vi "WW_Spin_Analysis_V2.vi"(11 "路径":path) -> (3 "strArrayError":string[](array[string]))   [LabVIEW 2011]
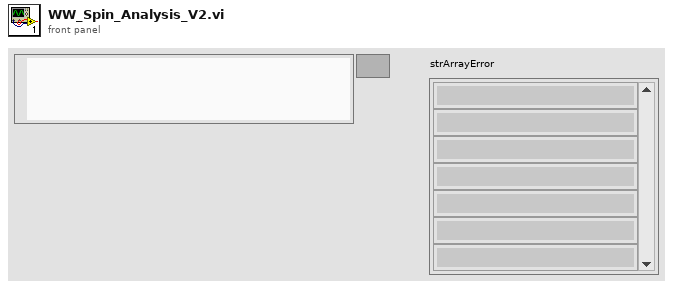
[diagram p1: front panel]
types:
  T1 = enum16{"RealTime", "WaterLevel", "WaterTemp", "AirTemp", "IPMTemp", "MotorActualRPM", "MotorTargetRPM", "FanActualRPM", "MemsSensorA", "MemsSensorB", "MemsSensorC", "WaterThermistorADC", "TouchSensor", "LeakageSensor", "DCLink", "IsDoorOpen", "IsTimeShort", "Progress", "Step", "TotalRemainTime", "StepRemainTime", "WeightSensingLowData", "WeightSensingResult", "ColdValve", "HotValve", "PreValve", "WaterShotValve", "BleachValve", "DryValve", "SteamValve", "SoftenerValve", "FilterValve", "IsDoorLocked", "SSRCommon", "MainRelay", "ACTUATOR2", "WaterDrainer", "CirculationPump", "WaterHeater", "DryHeater", "SteamHeater", "MotorDriveDirection", "IsDoubleDoorOpen", "IsDoubleDoorLock", "RunStateID", "PowerStateID", "SoundID", "ErrorCode", "OptionData", "MainVersion", "SUBVersion", "InverterVersion"}
  T2 = cluster{"mu32DrainIndex":u32, "mu32SpinIndex":u32, "mu32LooseInex":u32}
  T3 = cluster{"DrainTime":u32, "FinalSpinTime":u32, "LooseTime":u32, "SubTotalTime":u32}
  T4 = cluster{"Step1":cluster{"Speed":u32, "Time":u32}, "Step2":cluster{"Speed":u32, "Time":u32}, "Step3":cluster{"Speed":u32, "Time":u32}, "Untangle":cluster{"Speed":u32, "On":u32, "Off":u32}}
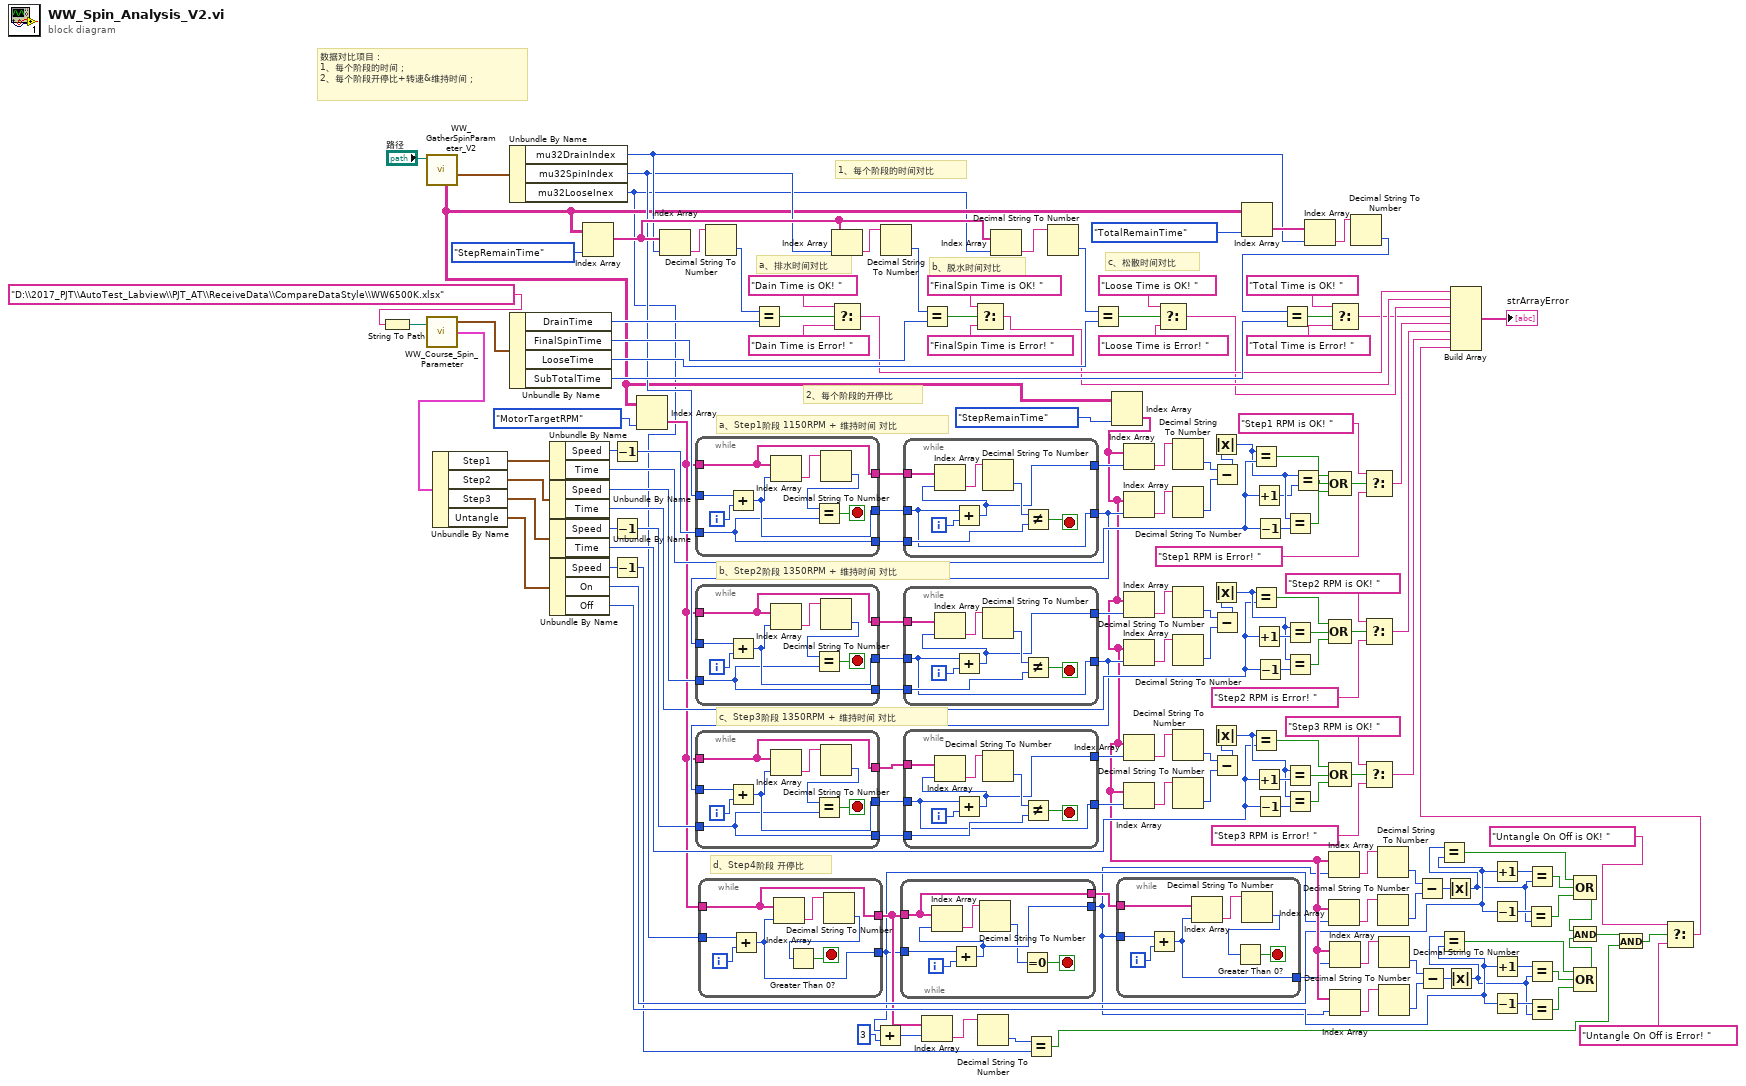
[diagram p0: block diagram]
diagram:
  # "d、Step4阶段 开停比"
  # "c、Step3阶段 1350RPM + 维持时间 对比"
  # "b、Step2阶段 1350RPM + 维持时间 对比"
  # "a、Step1阶段 1150RPM + 维持时间 对比"
  # "2、每个阶段的开停比"
  # "c、松散时间对比"
  # "b、脱水时间对比"
  # "a、排水时间对比"
  # "1、每个阶段的时间对比"
  # "数据对比项目：\n1、每个阶段的时间；\n2、每个阶段开停比+转速&维持时间；"
  n1 = String To Path(string="D:\\2017_PJT\\AutoTest_Labview\\PJT_AT\\ReceiveData\\CompareDataStyle\\WW6500K.xlsx") -> (path=w157:path)
  n2 = call "WW_GatherSpinParameter_V2.vi"("路径"="路径") -> ("strFinalSpinStepIndex"=w159:T2, "EXCEL读取"=w111:string[][])  [unwired: 4 in, 5 out]
  n3 = call "WW_Course_Spin_Parameter.vi"("路径"=w157) -> ("PrjFinalSpinTime"=w156:T3, "SpeedTime"=w123:T4)  [unwired: 1 in, 1 out]
  n4 = Unbundle By Name(w123) -> ("Step1"=w122:cluster{"Speed":u32, "Time":u32}, "Step2"=w121:cluster{"Speed":u32, "Time":u32}, "Step3"=w120:cluster{"Speed":u32, "Time":u32}, "Untangle"=w119:cluster{"Speed":u32, "On":u32, "Off":u32})
  n5 = Unbundle By Name(w159) -> ("mu32DrainIndex"=w135:u32, "mu32SpinIndex"=w117:u32, "mu32LooseInex"=w47:u32)
  n6 = Unbundle By Name(w156) -> ("DrainTime"=w155:u32, "FinalSpinTime"=w151:u32, "LooseTime"=w148:u32, "SubTotalTime"=w131:u32)
  n7 = Unbundle By Name(w122) -> ("Speed"=w114:u32, "Time"=w103:u32)
  n8 = Unbundle By Name(w121) -> ("Speed"=w73:u32, "Time"=w74:u32)
  n9 = Unbundle By Name(w120) -> ("Speed"=w50:u32, "Time"=w52:u32)
  n10 = Unbundle By Name(w119) -> ("Speed"=w49:u32, "On"=w33:u32, "Off"=w32:u32)
  n11 = Index Array(array=w111, index (col)=T1."StepRemainTime" ("WW_ParameterData")) -> (element=w147:string[])  [unwired: 1 in]
  n12 = Decrement(x=w114) -> (x-1=w113:u32)
  n13 = Decrement(x=w50) -> (x-1=w51:u32)
  n14 = Decrement(x=w49) -> (x-1=w5:u32)
  n15 = Index Array(array=w111, index (col)=T1."MotorTargetRPM" ("WW_ParameterData")) -> (element=w48:string[])  [unwired: 1 in]
  n16 = Index Array(array=w147, index=w135) -> (element=w160:string)
  n17 = while {
    tunnel: w48 -> [w164]
    tunnel: w117 -> [w169]
    tunnel: [w165] -> w116
    tunnel: [w164] -> w115
    tunnel: w113 -> [w163]
    tunnel: [w163] -> w112
    i -> [w170]
    stop <- w166 stop-if-true
    n18 = Add(x=w169, y=w170) -> (x+y=w165:u32)
    n19 = Index Array(array=w164, index=w165) -> (element=w168:string)
    n20 = Decimal String To Number(string=w168) -> (number=w167:i32)  [unwired: 2 in, 1 out]
    n21 = Equal?(x=w167, y=w163) -> (x = y?=w166:bool)
  }
  n22 = while {
    tunnel: w48 -> [w173]
    tunnel: w47 -> [w176]
    tunnel: [w174] -> w9
    tunnel: [w173] -> w11
    i -> [w177]
    stop <- w172 stop-if-true
    n23 = Add(x=w176, y=w177) -> (x+y=w174:u32)
    n24 = Index Array(array=w173, index=w174) -> (element=w175:string)
    n25 = Decimal String To Number(string=w175) -> (number=w171:i32)  [unwired: 2 in, 1 out]
    n26 = Greater Than 0?(x=w171) -> (x > 0?=w172:bool)
  }
  n27 = Decimal String To Number(string=w160) -> (number=w154:i32)  [unwired: 2 in, 1 out]
  n28 = Equal?(x=w154, y=w155) -> (x = y?=w153:bool)
  n29 = Index Array(array=w147, index=w117) -> (element=w152:string)
  n30 = Select(t="Dain Time is OK! ", s=w153, f="Dain Time is Error! ") -> (s? t:f=w128:string)
  n31 = Add(x=w9, y=u32 3) -> (x+y=w7:u32)
  n32 = Decimal String To Number(string=w152) -> (number=w150:i32)  [unwired: 2 in, 1 out]
  n33 = while {
    tunnel: w9 -> [w181]
    tunnel: w11 -> [w180]
    tunnel: [w182] -> w1
    tunnel: [w180] -> w46
    i -> [w183]
    stop <- w179 stop-if-true
    n34 = Add(x=w181, y=w183) -> (x+y=w182:u32)
    n35 = Index Array(array=w180, index=w182) -> (element=w184:string)
    n36 = Decimal String To Number(string=w184) -> (number=w178:i32)  [unwired: 2 in, 1 out]
    n37 = Equal To 0?(x=w178) -> (x = 0?=w179:bool)
  }
  n38 = while {
    tunnel: w116 -> [w185]
    tunnel: w115 -> [w192]
    tunnel: w112 -> [w187]
    tunnel: [w186] -> w107
    tunnel: [w185] -> w76
    i -> [w190]
    stop <- w188 stop-if-true
    n39 = Add(x=w185, y=w190) -> (x+y=w186:u32)
    n40 = Index Array(array=w192, index=w186) -> (element=w191:string)
    n41 = Decimal String To Number(string=w191) -> (number=w189:i32)  [unwired: 2 in, 1 out]
    n42 = Not Equal?(x=w189, y=w187) -> (x != y?=w188:bool)
  }
  n43 = while {
    tunnel: w48 -> [w194]
    tunnel: w76 -> [w199]
    tunnel: [w195] -> w94
    tunnel: [w194] -> w93
    tunnel: w73 -> [w193]
    tunnel: [w193] -> w92
    i -> [w200]
    stop <- w196 stop-if-true
    n44 = Add(x=w199, y=w200) -> (x+y=w195:u32)
    n45 = Index Array(array=w194, index=w195) -> (element=w198:string)
    n46 = Decimal String To Number(string=w198) -> (number=w197:i32)  [unwired: 2 in, 1 out]
    n47 = Equal?(x=w197, y=w193) -> (x = y?=w196:bool)
  }
  n48 = while {
    tunnel: w94 -> [w201]
    tunnel: w93 -> [w208]
    tunnel: w92 -> [w203]
    tunnel: [w202] -> w89
    tunnel: [w201] -> w53
    i -> [w206]
    stop <- w204 stop-if-true
    n49 = Add(x=w201, y=w206) -> (x+y=w202:u32)
    n50 = Index Array(array=w208, index=w202) -> (element=w207:string)
    n51 = Decimal String To Number(string=w207) -> (number=w205:i32)  [unwired: 2 in, 1 out]
    n52 = Not Equal?(x=w205, y=w203) -> (x != y?=w204:bool)
  }
  n53 = while {
    tunnel: w48 -> [w210]
    tunnel: w53 -> [w215]
    tunnel: [w211] -> w72
    tunnel: [w210] -> w71
    tunnel: w51 -> [w209]
    tunnel: [w209] -> w70
    i -> [w216]
    stop <- w212 stop-if-true
    n54 = Add(x=w215, y=w216) -> (x+y=w211:u32)
    n55 = Index Array(array=w210, index=w211) -> (element=w214:string)
    n56 = Decimal String To Number(string=w214) -> (number=w213:i32)  [unwired: 2 in, 1 out]
    n57 = Equal?(x=w213, y=w209) -> (x = y?=w212:bool)
  }
  n58 = while {
    tunnel: w72 -> [w217]
    tunnel: w71 -> [w224]
    tunnel: w70 -> [w219]
    tunnel: [w218] -> w67
    tunnel: [w217] -> w66
    i -> [w222]
    stop <- w220 stop-if-true
    n59 = Add(x=w217, y=w222) -> (x+y=w218:u32)
    n60 = Index Array(array=w224, index=w218) -> (element=w223:string)
    n61 = Decimal String To Number(string=w223) -> (number=w221:i32)  [unwired: 2 in, 1 out]
    n62 = Not Equal?(x=w221, y=w219) -> (x != y?=w220:bool)
  }
  n63 = Equal?(x=w150, y=w151) -> (x = y?=w149:bool)
  n64 = Index Array(array=w11, index=w7) -> (element=w10:string)
  n65 = Select(t="FinalSpin Time is OK! ", s=w149, f="FinalSpin Time is Error! ") -> (s? t:f=w127:string)
  n66 = Decimal String To Number(string=w10) -> (number=w6:i32)  [unwired: 2 in, 1 out]
  n67 = Index Array(array=w147, index=w47) -> (element=w146:string)
  n68 = Equal?(x=w6, y=w5) -> (x = y?=w3:bool)
  n69 = Decimal String To Number(string=w146) -> (number=w145:i32)  [unwired: 2 in, 1 out]
  n70 = Equal?(x=w145, y=w148) -> (x = y?=w144:bool)
  n71 = Index Array(array=w111, index (col)=T1."StepRemainTime" ("WW_ParameterData")) -> (element=w35:string[])  [unwired: 1 in]
  n72 = while {
    tunnel: w46 -> [w225]
    tunnel: w1 -> [w230]
    tunnel: [w226] -> w34
    i -> [w231]
    stop <- w227 stop-if-true
    n73 = Add(x=w230, y=w231) -> (x+y=w226:u32)
    n74 = Index Array(array=w225, index=w226) -> (element=w229:string)
    n75 = Decimal String To Number(string=w229) -> (number=w228:i32)  [unwired: 2 in, 1 out]
    n76 = Greater Than 0?(x=w228) -> (x > 0?=w227:bool)
  }
  n77 = Index Array(array=w35, index=w107) -> (element=w109:string)
  n78 = Index Array(array=w35, index=w76) -> (element=w108:string)
  n79 = Index Array(array=w35, index=w89) -> (element=w91:string)
  n80 = Index Array(array=w35, index=w53) -> (element=w90:string)
  n81 = Index Array(array=w35, index=w67) -> (element=w69:string)
  n82 = Index Array(array=w35, index=w66) -> (element=w68:string)
  n83 = Select(t="Loose Time is OK! ", s=w144, f="Loose Time is Error! ") -> (s? t:f=w126:string)
  n84 = Decimal String To Number(string=w109) -> (number=w106:i32)  [unwired: 2 in, 1 out]
  n85 = Decimal String To Number(string=w108) -> (number=w105:i32)  [unwired: 2 in, 1 out]
  n86 = Decimal String To Number(string=w91) -> (number=w88:i32)  [unwired: 2 in, 1 out]
  n87 = Decimal String To Number(string=w90) -> (number=w87:i32)  [unwired: 2 in, 1 out]
  n88 = Decimal String To Number(string=w69) -> (number=w65:i32)  [unwired: 2 in, 1 out]
  n89 = Decimal String To Number(string=w68) -> (number=w64:i32)  [unwired: 2 in, 1 out]
  n90 = Subtract(x=w106, y=w105) -> (x-y=w104:i32)
  n91 = Absolute Value(x=w104) -> (abs(x)=w101:i32)
  n92 = Subtract(x=w88, y=w87) -> (x-y=w86:i32)
  n93 = Absolute Value(x=w86) -> (abs(x)=w83:i32)
  n94 = Subtract(x=w65, y=w64) -> (x-y=w63:i32)
  n95 = Absolute Value(x=w63) -> (abs(x)=w60:i32)
  n96 = Index Array(array=w111, index (col)=T1."TotalRemainTime" ("WW_ParameterData")) -> (element=w136:string[])  [unwired: 1 in]
  n97 = Equal?(x=w101, y=w103) -> (x = y?=w100:bool)
  n98 = Equal?(x=w83, y=w74) -> (x = y?=w82:bool)
  n99 = Equal?(x=w60, y=w52) -> (x = y?=w59:bool)
  n100 = Increment(x=w103) -> (x+1=w75:u32)
  n101 = Increment(x=w74) -> (x+1=w85:u32)
  n102 = Increment(x=w52) -> (x+1=w62:u32)
  n103 = Decrement(x=w103) -> (x-1=w102:u32)
  n104 = Decrement(x=w74) -> (x-1=w84:u32)
  n105 = Decrement(x=w52) -> (x-1=w61:u32)
  n106 = Equal?(x=w101, y=w102) -> (x = y?=w98:bool)
  n107 = Equal?(x=w83, y=w85) -> (x = y?=w81:bool)
  n108 = Equal?(x=w83, y=w84) -> (x = y?=w80:bool)
  n109 = Equal?(x=w60, y=w62) -> (x = y?=w58:bool)
  n110 = Equal?(x=w60, y=w61) -> (x = y?=w57:bool)
  n111 = Equal?(x=w101, y=w75) -> (x = y?=w99:bool)
  n112 = Index Array(array=w136, index=w135) -> (element=w134:string)
  n113 = Compound Arithmetic op=OR(w100, w99, w98) -> (w97:bool)
  n114 = Compound Arithmetic op=OR(w82, w81, w80) -> (w79:bool)
  n115 = Compound Arithmetic op=OR(w59, w58, w57) -> (w56:bool)
  n116 = Index Array(array=w35, index=w1) -> (element=w45:string)
  n117 = Index Array(array=w35, index=w9) -> (element=w44:string)
  n118 = Index Array(array=w35, index=w34) -> (element=w40:string)
  n119 = Index Array(array=w35, index=w1) -> (element=w39:string)
  n120 = Decimal String To Number(string=w134) -> (number=w132:i32)  [unwired: 2 in, 1 out]
  n121 = Equal?(x=w132, y=w131) -> (x = y?=w133:bool)
  n122 = Select(t="Total Time is OK! ", s=w133, f="Total Time is Error! ") -> (s? t:f=w125:string)
  n123 = Select(t="Step1 RPM is OK! ", s=w97, f="Step1 RPM is Error! ") -> (s? t:f=w15:string)
  n124 = Select(t="Step2 RPM is OK! ", s=w79, f="Step2 RPM is Error! ") -> (s? t:f=w14:string)
  n125 = Select(t="Step3 RPM is OK! ", s=w56, f="Step3 RPM is Error! ") -> (s? t:f=w13:string)
  n126 = Decimal String To Number(string=w45) -> (number=w43:i32)  [unwired: 2 in, 1 out]
  n127 = Decimal String To Number(string=w44) -> (number=w42:i32)  [unwired: 2 in, 1 out]
  n128 = Decimal String To Number(string=w40) -> (number=w38:i32)  [unwired: 2 in, 1 out]
  n129 = Decimal String To Number(string=w39) -> (number=w37:i32)  [unwired: 2 in, 1 out]
  n130 = Subtract(x=w43, y=w42) -> (x-y=w41:i32)
  n131 = Subtract(x=w38, y=w37) -> (x-y=w36:i32)
  n132 = Absolute Value(x=w41) -> (abs(x)=w28:i32)
  n133 = Equal?(x=w28, y=w33) -> (x = y?=w25:bool)
  n134 = Absolute Value(x=w36) -> (abs(x)=w26:i32)
  n135 = Equal?(x=w26, y=w32) -> (x = y?=w22:bool)
  n136 = Increment(x=w33) -> (x+1=w31:u32)
  n137 = Decrement(x=w33) -> (x-1=w30:u32)
  n138 = Increment(x=w32) -> (x+1=w29:u32)
  n139 = Decrement(x=w32) -> (x-1=w27:u32)
  n140 = Equal?(x=w30, y=w28) -> (x = y?=w23:bool)
  n141 = Equal?(x=w31, y=w28) -> (x = y?=w24:bool)
  n142 = Equal?(x=w29, y=w26) -> (x = y?=w21:bool)
  n143 = Equal?(x=w27, y=w26) -> (x = y?=w20:bool)
  n144 = Compound Arithmetic op=OR(w25, w24, w23) -> (w19:bool)
  n145 = Compound Arithmetic op=OR(w22, w21, w20) -> (w18:bool)
  n146 = And(x=w19, y=w18) -> (x .and. y?=w4:bool)
  n147 = And(x=w4, y=w3) -> (x .and. y?=w2:bool)
  n148 = Select(t="Untangle On Off is OK! ", s=w2, f="Untangle On Off is Error! ") -> (s? t:f=w12:string)
  n149 = Build Array(w128, w127, w126, w125, w15, w14, w13, w12) -> (→"strArrayError":string[])
